vi "NT Read Boolean Array.vi"(4 "options":T1={"Send All"=FALSE, "Keep Duplicates"=FALSE, "rate (hz)"=10}, 8 "error in":errorcluster, 9 "default value":bool[](array[boolean]), 11 "name":string="Boolean Array") -> (0 "error out":errorcluster, 1 "timestamp":u64, 3 "value":bool[](array[boolean]))   [LabVIEW 2025]
doc: "Return the Boolean array data stored in the named topic. Returns an error and the default value if topic not present."
uses:
  <vilib>/Rock Robotics/Network Tables/NT SubscribeOptions.ctl
  <vilib>/Rock Robotics/Network Tables/NT Datatype.ctl
panel:
  in  "description":string="boolean[]"
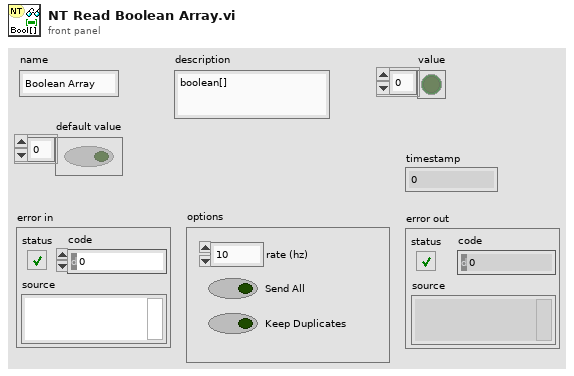
[diagram p1: front panel]
types:
  T1 = typedef "NT SubscribeOptions.ctl" = cluster{"Send All":bool, "Keep Duplicates":bool, "rate (hz)":u64}
  T2 = typedef "NT Datatype.ctl" = u32
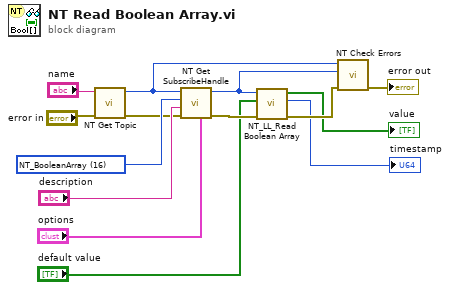
[diagram p0: block diagram]
diagram:
  w10 = T2 16 items=["NT_Unassigned"=0, "NT_Boolean"=1, "NT_Double"=2, "NT_String"=4, "NT_Raw"=8, "NT_BooleanArray"=16, "NT_DoubleArray"=32, "NT_StringArray"=64, "NT_RPC"=128, "NT_Integer"=256, "NT_Float"=512, "NT_IntegerArray"=1024, "NT_FloatArray"=2048] ("NT_Type")
  n1 = call <vilib>:"NT Get Topic.vi"("error in (no error)"="error in", "name"="name") -> ("error out"=w9:errorcluster, "topicHandle"=w6:u32)  [unwired: 8 in]
  n2 = call <vilib>:"NT Get SubscribeHandle.vi"("options"="options", "error in (no error)"=w9, "description"="description", "NT_Type"=w10, "topicHandle"=w6) -> ("error out"=w8:errorcluster, "subscribeHandle"=w1:u32)  [unwired: 5 in]
  n3 = call <vilib>:"NT_LL_Read Boolean Array.vi"("error in (no error)"=w8, "default value"="default value", "subscribeHandle"=w1) -> ("error out"=w7:errorcluster, "time"=→"timestamp":i64, "value"=→"value":bool[])  [unwired: 5 in, 1 out]
  n4 = call <vilib>:"NT Check Errors.vi"("error in (no error)"=w7, "pubSubHandle"=w1, "topicHandle"=w6) -> ("error out"=→"error out":errorcluster)  [unwired: 8 in]
